vi "Data_analyzer.vi"(8 "error in":errorcluster, 10 "Vsupni cluster":T1 {"Hystereze" min=0.0 step=0.1}, 11 "Data":waveform(dbl)) -> (0 "error out":errorcluster, 2 "Pocet period":i32, 3 "Prubeh frekvence":waveform(dbl))   [LabVIEW 2021]
uses:
  Vstupni_cluster.ctl
  Stavy_Data_analyzer.ctl
  <vilib>/Waveform/WDTOps.llb/WDT Get Waveform Time Array DBL.vi
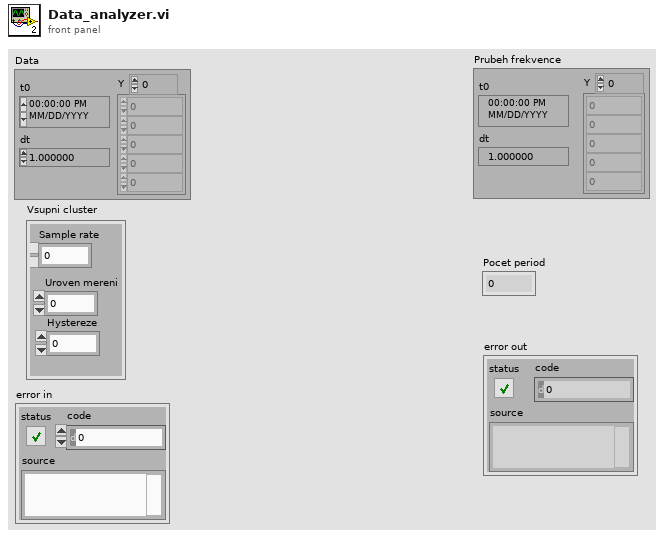
[diagram p1: front panel]
types:
  T1 = typedef "Vstupni_cluster.ctl" = cluster{"Uroven mereni":dbl, "Hystereze":dbl, "Sample rate":dbl}
  T2 = typedef "Stavy_Data_analyzer.ctl" = enum16{"Pociatok", "Detekce vzestupne - kladna", "Detekce vzestupne - zaporna", "Detekce sestupne - kladna", "Detekce sestupne - zaporna"}
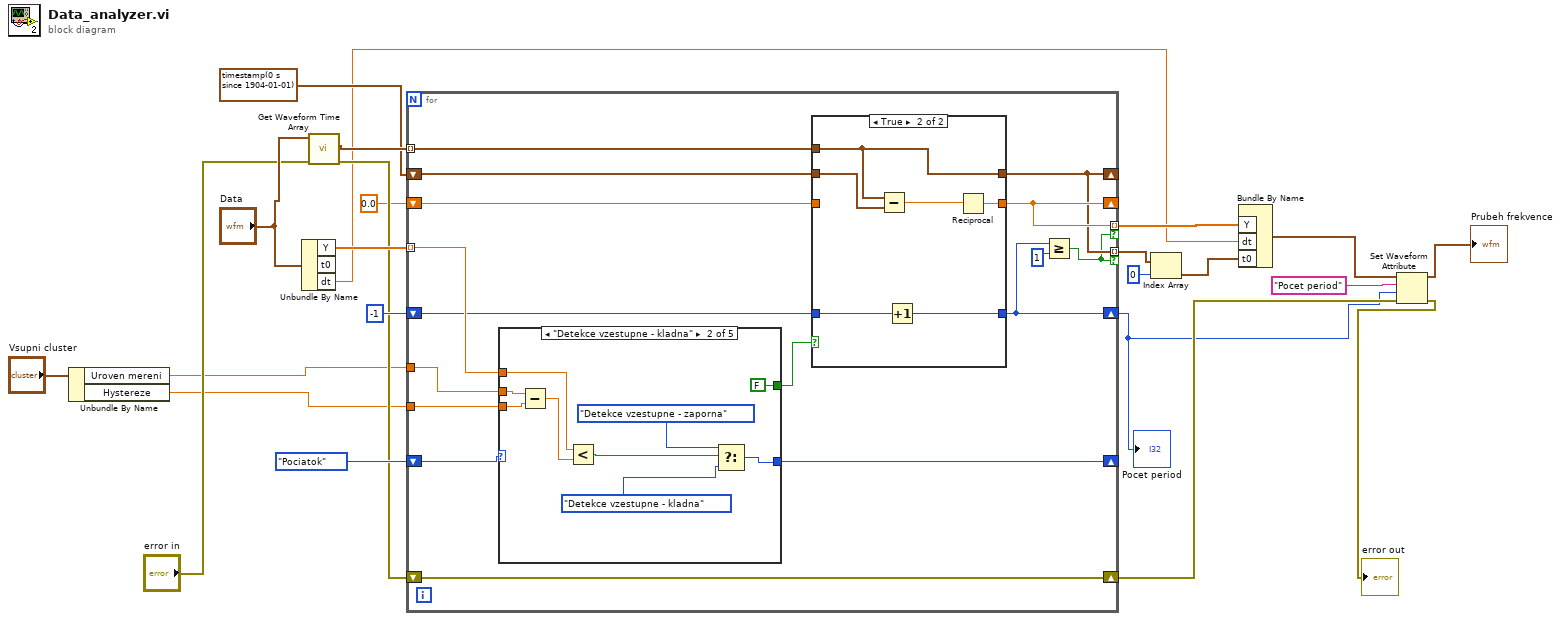
[diagram p0: block diagram]
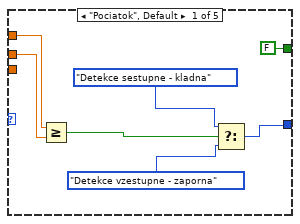
[diagram p3: hidden frame]
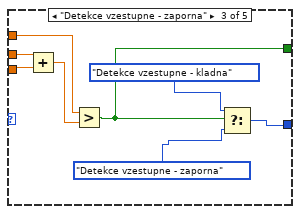
[diagram p4: hidden frame]
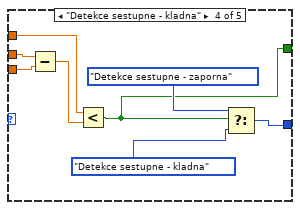
[diagram p5: hidden frame]
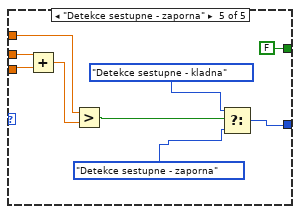
[diagram p6: hidden frame]
diagram:
  n1 = Unbundle By Name("Vsupni cluster") -> ("Uroven mereni"=w9:dbl, "Hystereze"=w8:dbl)
  n2 = Unbundle By Name("Data") -> ("Y"=w23:dbl[], "dt"=w13:dbl)  [unwired: 1 out]
  n3 = call-poly <vilib>:"Get Waveform Time Array.vi"("error in (no error)"="error in", "waveform in"="Data") -> ("error out"=w19:errorcluster, "X array"=w17:timestamp[])  [unwired: 8 in]
  n4 = for {
    tunnel: w23 -> [w37] mode=indexing
    tunnel: w9 -> [w38]
    shift-right: [w32] -> w7
    shift-left: w19 -> [w32]
    tunnel: w8 -> [w39]
    shift-right: [w35] -> _
    shift-left: Stavy_Data_analyzer."Pociatok" -> [w36]
    shift-right: [w27] -> w1
    shift-left: -1 -> [w34]
    tunnel: w17 -> [w33] mode=indexing
    shift-right: [w25] -> _
    shift-left: timestamp(0 s since 1904-01-01) ("element") -> [w31]
    shift-right: [w28] -> _
    shift-left: 0.0 -> [w29]
    tunnel: [w28] -> w14 mode=indexing if=w24
    tunnel: [w25] -> w12 mode=indexing if=w24
    n5 = case shown="\"Detekce vzestupne - kladna\"" w36 {
      tunnel: w39 -> [_ w63 w69 w79 w86]
      tunnel: w38 -> [w54 w62 w70 w78 w87]
      tunnel: w37 -> [w55 w61 w71 w77 w88]
      tunnel: [w52 w60 w68 w76 w85] -> w35
      tunnel: [FALSE FALSE w67 w73 FALSE] -> w30
      frame "Pociatok", Default {
        n6 = Greater Or Equal?(x=w55, y=w54) -> (x >= y?=w53:bool)
        n7 = Select(t=Stavy_Data_analyzer."Detekce sestupne - kladna", s=w53, f=Stavy_Data_analyzer."Detekce vzestupne - zaporna") -> (s? t:f=w52:T2)
      }
      frame "Detekce vzestupne - kladna" {
        n8 = Subtract(x=w62, y=w63) -> (x-y=w64:dbl)
        n9 = Less?(x=w61, y=w64) -> (x < y?=w59:bool)
        n10 = Select(t=Stavy_Data_analyzer."Detekce vzestupne - zaporna", s=w59, f=Stavy_Data_analyzer."Detekce vzestupne - kladna") -> (s? t:f=w60:T2)
      }
      frame "Detekce vzestupne - zaporna" {
        n11 = Add(x=w70, y=w69) -> (x+y=w72:dbl)
        n12 = Greater?(x=w71, y=w72) -> (0:w67:bool)
        n13 = Select(t=Stavy_Data_analyzer."Detekce vzestupne - kladna", s=w67, f=Stavy_Data_analyzer."Detekce vzestupne - zaporna") -> (s? t:f=w68:T2)
      }
      frame "Detekce sestupne - kladna" {
        n14 = Subtract(x=w78, y=w79) -> (x-y=w80:dbl)
        n15 = Less?(x=w77, y=w80) -> (x < y?=w73:bool)
        n16 = Select(t=Stavy_Data_analyzer."Detekce sestupne - zaporna", s=w73, f=Stavy_Data_analyzer."Detekce sestupne - kladna") -> (s? t:f=w76:T2)
      }
      frame "Detekce sestupne - zaporna" {
        n17 = Add(x=w87, y=w86) -> (x+y=w89:dbl)
        n18 = Greater?(x=w88, y=w89) -> (0:w84:bool)
        n19 = Select(t=Stavy_Data_analyzer."Detekce sestupne - kladna", s=w84, f=Stavy_Data_analyzer."Detekce sestupne - zaporna") -> (s? t:f=w85:T2)
      }
    }
    n20 = case shown="True" w30 {
      tunnel: w34 -> [w42 w48]
      tunnel: [w42 w47] -> w27
      tunnel: w33 -> [_ w44]
      tunnel: [w41 w44] -> w25
      tunnel: w31 -> [w41 w43]
      tunnel: [w40 w46] -> w28
      tunnel: w29 -> [w40 _]
      frame False {
      }
      frame True {
        n21 = Subtract(x=w44, y=w43) -> (x-y=w45:dbl)
        n22 = Increment(x=w48) -> (x+1=w47:i32)
        n23 = Reciprocal(x=w45) -> (1/x=w46:dbl)
      }
    }
    n24 = Greater Or Equal?(x=w27, y=1) -> (x >= y?=w24:bool)
  }
  "Pocet period" <- w1
  n25 = Index Array(array=w12, index=0) -> (element=w5:timestamp)
  n26 = Bundle By Name("Y"=w14, "dt"=w13, "t0"=w5) -> (w4:waveform(dbl))  [unwired: 1 in]
  n27 = Set Waveform Attribute(4:w7, 5:w1, 6:"Pocet period" ("name"), 7:w4) -> (0:→"error out":errorcluster, 3:→"Prubeh frekvence":waveform(dbl))  [unwired: 1 out]
